vi "PID (SubVI).vi"(8 "PID gains":cluster{"Kp":dbl, "Ki":dbl, "Kd":dbl}={"Kp"=0.01, "Ki"=0.0087, "Kd"=0.00011267}, 10 "Output":dbl, 11 "Ref":dbl) -> (3 "Control":dbl)   [LabVIEW 2016]
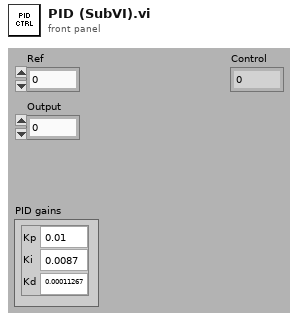
[diagram p1: front panel]
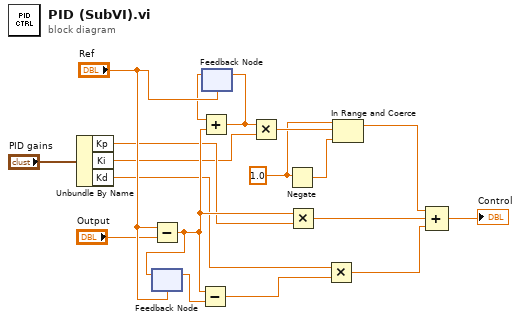
[diagram p0: block diagram]
diagram:
  w11 = 1.0 ("Windup Limit")
  n1 = Unbundle By Name("PID gains") -> ("Kp"=w9:dbl, "Ki"=w8:dbl, "Kd"=w7:dbl)
  n2 = Subtract(x="Ref", y="Output") -> (x-y=w17:dbl)
  n3 = feedback-in #1(w17) -> ()
  n4 = feedback #1("Ref") -> (w14:dbl)
  n5 = Subtract(x=w17, y=w14) -> (x-y=w13:dbl)
  n6 = feedback #2("Ref") -> (w15:dbl)
  n7 = Add(x=w15, y=w17) -> (x+y=w16:dbl)
  n8 = feedback-in #2(w16) -> ()
  n9 = Multiply(x=w16, y=w8) -> (x*y=w12:dbl)
  n10 = Negate(x=w11) -> (-x=w10:dbl)
  n11 = Multiply(x=w17, y=w9) -> (x*y=w4:dbl)
  n12 = Multiply(x=w7, y=w13) -> (x*y=w3:dbl)
  n13 = In Range and Coerce(upper limit=w11, x=w12, lower limit=w10) -> (coerced(x)=w2:dbl)  [unwired: 1 out]
  n14 = Compound Arithmetic op=ADD(w2, w4, w3) -> (→"Control":dbl)
